vi "All.vi"() -> ()   [LabVIEW 2013]
panel:
  in  "Transmitter Properties":T1 {"Window" items=["Rectangular", "Bohman", "Parzen", "Bartlett-Hanning", "Blackman-Nuttall", "Blackman", "Hanning", "Hamming", "Welch", "Exact Blackman", "Blackman-Harris", "Triangle"]}
  in  "Input Bits":bool[](array[boolean])
  out "Output Bits":bool[](array[boolean])
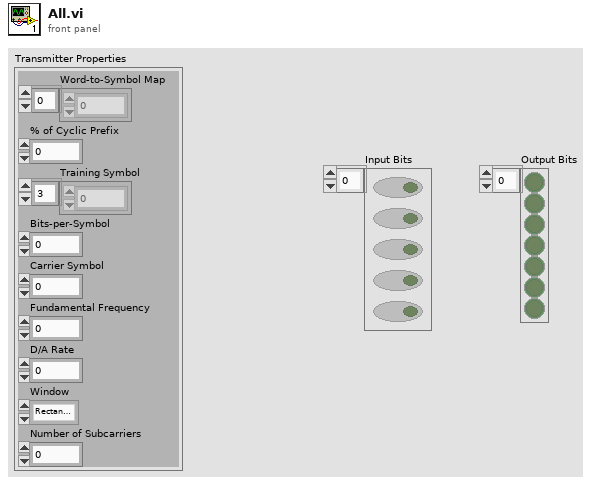
[diagram p1: front panel]
types:
  T1 = cluster{"Word-to-Symbol Map":cdb[], "% of Cyclic Prefix":dbl, "Training Symbol":cdb[], "Bits-per-Symbol":i32, "Carrier Symbol":cdb, "Fundamental Frequency":dbl, "D/A Rate":dbl, "Window":u16, "Number of Subcarriers":i32}
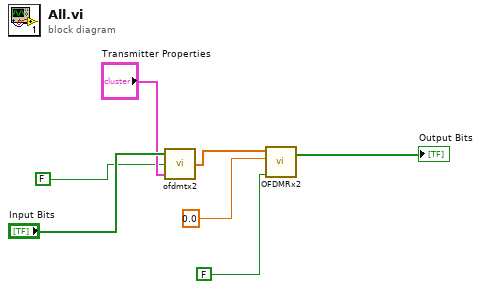
[diagram p0: block diagram]
diagram:
  n1 = call "ofdmtx2.vi"("Transmitter Properties"="Transmitter Properties", "Generate Training Symbol"=FALSE, "Input Bits"="Input Bits") -> ("OFDM Signal"=w3:cdb[])
  n2 = call "OFDMRx2.vi"("Input Signal"=w3, "Frequency Offset"=0.0, "Equalize"=FALSE) -> ("Output Bits"=→"Output Bits":bool[])  [unwired: 3 in]
